vi "Get Chat[ ].vi"(8 "error in (no error)":errorcluster, 11 "Telegram Class in":refnum<class "Telegram Class.lvclass">) -> (0 "error out":errorcluster, 2 "Chat[ ]":string[][](array[string]), 3 "Telegram Class out":refnum<class "Telegram Class.lvclass">)   [LabVIEW 2015, in "Telegram Library.lvlib" / "Telegram Class.lvclass"]
doc: "Created IvanLis by LabVIEW Portal\nProfile: http://labviewportal.org/memberlist.php?mode=viewprofile&u=987\neMail: IvanLisanov@gMail.com\nTelegram: https://t.me/IvanLis"
uses:
  Telegram Class.lvclass
  Telegram Class.lvclass/Telegram Class.ctl
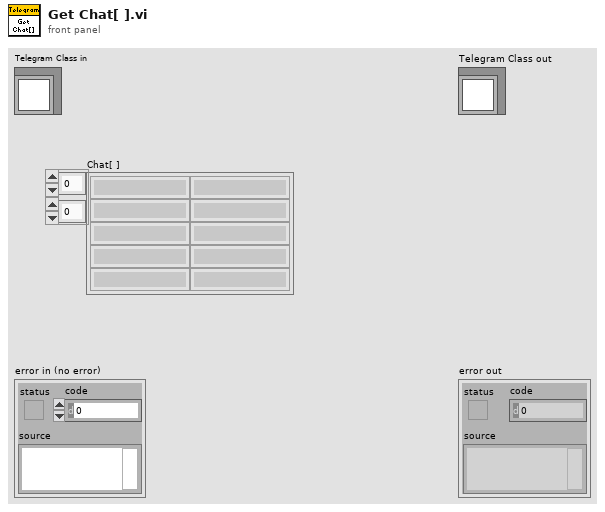
[diagram p1: front panel]
types:
  T1 = typedef "Telegram Library.lvlib/Chat.ctl" = cluster{"id":i64, "position":i64, "title":string}
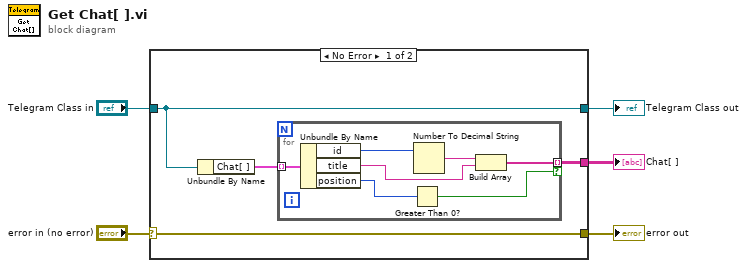
[diagram p0: block diagram]
diagram:
  n1 = case shown="No Error" "error in (no error)" {
    selector: "error in (no error)" -> [w6 w18]
    tunnel: [w6 w18] -> w4
    tunnel: [w7 w17] -> w2
    tunnel: "Telegram Class in" -> [w7 w17]
    tunnel: [w9 _] -> w1
    frame No Error {
      n2 = Unbundle By Name(w7) -> ("Chat[ ]"=w8:T1[])
      n3 = for {
        tunnel: w8 -> [w16] mode=indexing
        tunnel: [w14] -> w9 mode=indexing if=w10
        n4 = Unbundle By Name(w16) -> ("id"=w12:i64, "title"=w13:string, "position"=w11:i64)
        n5 = Greater Than 0?(x=w11) -> (x > 0?=w10:bool)
        n6 = Number To Decimal String(number=w12) -> (decimal integer string=w15:string)  [unwired: 1 in]
        n7 = Build Array(w15, w13) -> (w14:string[])
      }
    }
    frame Error {
    }
  }
  "error out" <- w4
  "Telegram Class out" <- w2
  "Chat[ ]" <- w1
